vi "K6221_SetPoint.vi"() -> ()   [LabVIEW 2018]
panel:
  out "Current Set Point (mA)":dbl format="%#_4g"
  in  "VISA resource name":refnum<visa-resource-name>="GPIB0::20::INSTR"
  in  "Current (mA)":dbl format="%#_4g"
  in  "Data mac ip address":string="146.201.201.70"
  in  "port":u16=3375
  in  "error in (no error)":errorcluster
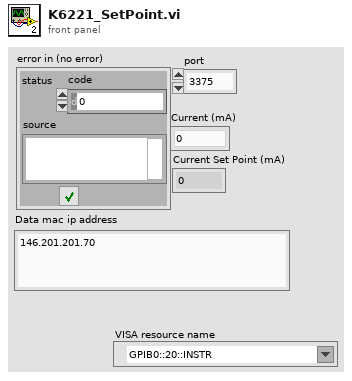
[diagram p1: front panel]
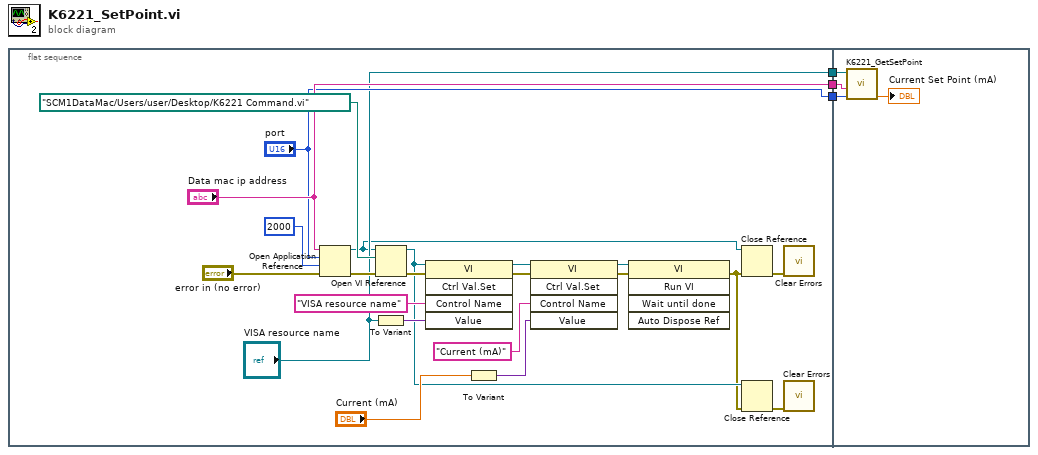
[diagram p0: block diagram]
diagram:
  n1 = flat-sequence {
    tunnel: ["Data mac ip address"] -> w3
    tunnel: ["port"] -> w2
    tunnel: ["VISA resource name"] -> w1
    tunnel: w3 -> [w28]
    tunnel: w2 -> [w27]
    tunnel: w1 -> [w26]
    frame #0 {
      n2 = Open Application Reference(8:"error in (no error)", 9:2000 ("timeout ms (60000)"), 10:"port", 11:"Data mac ip address") -> (0:w22:errorcluster, 3:w8:refnum<vi>)
      n3 = Open VI Reference(application reference (local)=w8, vi path=path "/SCM1DataMac/Users/user/Desktop/K6221 Command.vi", error in (no error)=w22) -> (vi reference=w7:refnum<vi>, error out=w21:errorcluster)  [unwired: 3 in]
      n4 = To Variant(anything="VISA resource name") -> (Variant=w19:variant)
      n5 = invoke class="VI" method="Ctrl Val.Set"(reference=w7, error in=w21, "Control Name"="VISA resource name", "Value"=w19) -> (reference out=w18:refnum<vi>, error out=w17:errorcluster)  [unwired: 1 in, 3 out]
      n6 = To Variant(anything="Current (mA)") -> (Variant=w14:variant)
      n7 = invoke class="VI" method="Ctrl Val.Set"(reference=w18, error in=w17, "Control Name"="Current (mA)", "Value"=w14) -> (reference out=w13:refnum<vi>, error out=w12:errorcluster)  [unwired: 1 in, 3 out]
      n8 = invoke class="VI" method="Run VI"(reference=w13, error in=w12) -> (error out=w4:errorcluster)  [unwired: 3 in, 4 out]
      n9 = Close Reference(reference=w8, error in (no error)=w4) -> (error out=w5:errorcluster)
      n10 = Close Reference(reference=w7, error in (no error)=w4) -> (error out=w6:errorcluster)
      n11 = call <vilib>:"Clear Errors.vi"("error in (no error)"=w5) -> ()  [unwired: 5 in, 2 out]
      n12 = call <vilib>:"Clear Errors.vi"("error in (no error)"=w6) -> ()  [unwired: 5 in, 2 out]
    }
    frame #1 {
      n13 = call "K6221_GetSetPoint.vi"("port"=w27, "Data mac ip address"=w28, "VISA resource name"=w26) -> ("Current Set Point (mA)"=→"Current Set Point (mA)":dbl)  [unwired: 7 in, 1 out]
    }
  }
